vi "Drive Immediate.vi"(6 "Straight Setpoint":dbl, 7 "Description":string, 8 "Command Info In":T1, 9 "Deadband Value":dbl=0.01, 10 "Right Setpoint":dbl, 11 "Left Setpoint":dbl) -> (0 "Command Info Out":T1)   [LabVIEW 2015]
doc: "Often used for joystick control, this VI checks to see that the joystick axes are outside the deadband and updates the motors appropriately."
uses:
  <vilib>/Rock Robotics/WPI/Framework/Command Status Info.ctl
  <vilib>/Rock Robotics/WPI/Framework/Completion Status.ctl
  <vilib>/Rock Robotics/WPI/Framework/Completion Notifier.ctl
  Implementation/Drive Setpoints.ctl
  Implementation/Drive Operations.ctl
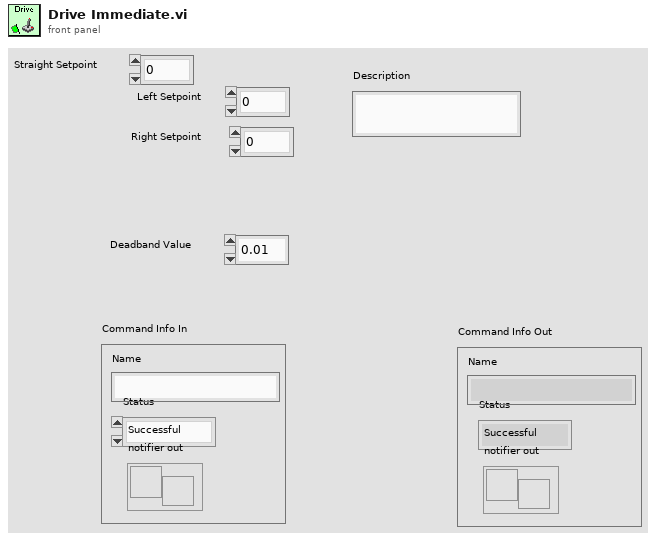
[diagram p1: front panel]
types:
  T1 = typedef "Command Status Info.ctl" = cluster{"Name":string, "Status":T2, "notifier out":T3}
  T2 = typedef "Completion Status.ctl" = enum16{"Successful", "Aborted", "Incomplete"}
  T3 = typedef "Completion Notifier.ctl" = refnum<notifier>
  T4 = typedef "Drive Setpoints.ctl" = cluster{"Operation":T5, "Left Setpoint":dbl, "Right Setpoint":dbl, "Duration":dbl, "Position":cluster{"X":dbl, "Y":dbl, "Angle":dbl, "Distance":dbl}, "Straight Setpoint":dbl}
  T5 = typedef "Drive Operations.ctl" = enum16{"Reserve", "Read Current", "Immediate", "Turn to Angle", "Pick Up Ball", "Drive Straight", "Drive to Target (arc)"}
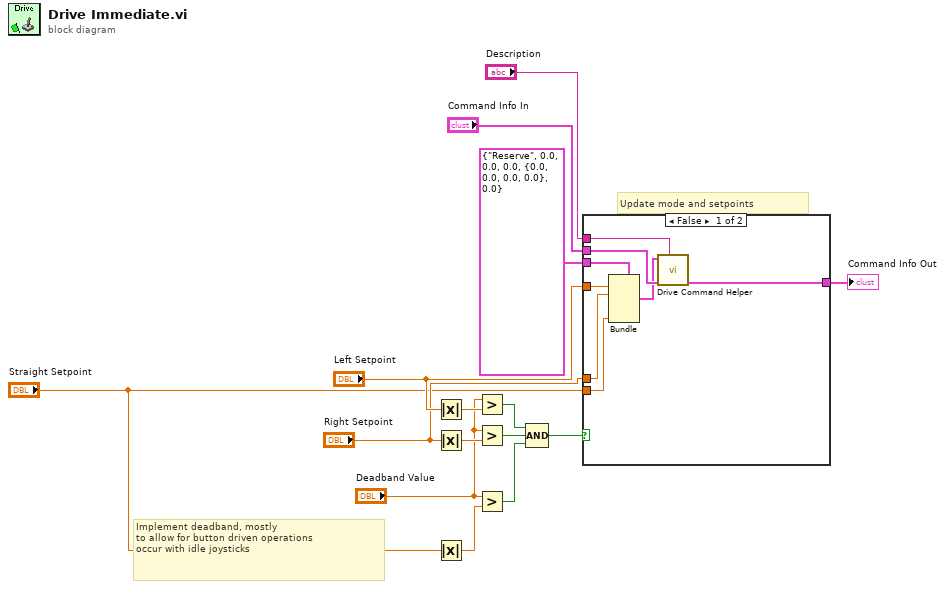
[diagram p0: block diagram]
diagram:
  # "Implement deadband, mostly\nto allow for button driven operations\noccur with idle joysticks"
  # "Update mode and setpoints"
  n1 = Absolute Value(x="Left Setpoint") -> (abs(x)=w15:dbl)
  n2 = Absolute Value(x="Right Setpoint") -> (abs(x)=w10:dbl)
  n3 = Absolute Value(x="Straight Setpoint") -> (abs(x)=w5:dbl)
  n4 = Greater?(x="Deadband Value", y=w15) -> (0:w8:bool)
  n5 = Greater?(x="Deadband Value", y=w10) -> (0:w7:bool)
  n6 = Greater?(x="Deadband Value", y=w5) -> (0:w3:bool)
  n7 = Compound Arithmetic op=AND(w8, w7, w3) -> (w2:bool)
  n8 = case shown="False" w2 {
    tunnel: "Left Setpoint" -> [w23 _]
    tunnel: T4 {"Operation"=enum."Reserve", "Left Setpoint"=0.0, "Right Setpoint"=0.0, "Duration"=0.0, "Position"={"X"=0.0, "Y"=0.0, "Angle"=0.0, "Distance"=0.0}, "Straight Setpoint"=0.0} ("SubSystem Data") -> [w22 _]
    tunnel: [w21 w24] -> w14
    tunnel: "Command Info In" -> [w20 w24]
    tunnel: "Description" -> [w19 _]
    tunnel: "Right Setpoint" -> [w18 _]
    tunnel: "Straight Setpoint" -> [w16 _]
    frame False {
      n9 = Bundle(cluster=w22, "Left Setpoint"=w23, "Right Setpoint"=w18, "Straight Setpoint"=w16) -> (w17:T4)  [unwired: 3 in]
      n10 = call "Drive Command Helper.vi"("Description"=w19, "Command Info In"=w20, "SubSystem Data"=w17) -> ("Command Info Out"=w21:T1)  [unwired: 7 in, 1 out]
    }
    frame True {
    }
  }
  "Command Info Out" <- w14
